vi "Main-loop.vi"() -> ()   [LabVIEW 2016]
uses:
  Sched_state.ctl
  Plant_info.ctl
  <vilib>/Platform/TimedLoop/XDataNode/timing_clust.ctl
  <vilib>/Platform/TimedLoop/XDataNode/nitl_modes.ctl
  <vilib>/Platform/TimedLoop/XDataNode/wakeup.ctl
  <vilib>/Platform/TimedLoop/XDataNode/XDataNode.xnode
  <vilib>/Platform/TimedLoop/XDataNode/XDNodeRunTimeDep.lvlib
panel:
  in  "Machine 1 IP Address":string="193.0.0.2"
  in  "Machine 2 IP address":string="193.0.0.4"
  in  "Plant 2 VI path":path=path "C:/ni-rt/startup/Plant2.vi"
  in  "Plant 1 VI path":path=path "C:/ni-rt/startup/Plant1.vi"
  out "error out":errorcluster
  out "loop time\n(only for diagnostics) - should be exactly 10, always":u32
  out "Plant 2 region":dbl(graph)
  out "Plant 1 region":dbl(graph)
  out "Plant 2":cluster{"Input":dbl, "Data":dbl, "Data":dbl}(graph)
  out "Plant 1":cluster{"Input":dbl, "Data":dbl, "Data":dbl}(graph)
  in  "error in (no error)":errorcluster
  in  "stop main":bool
  # "IMPORTANT! Deploy all files on the PXI machines in which the plants reside (Right-click on the target in the project > Deploy All) before starting this VI"
  # "Note that the \"VI paths\" for the plants refer to paths in the context of the respective PXI machines. not on this machine"
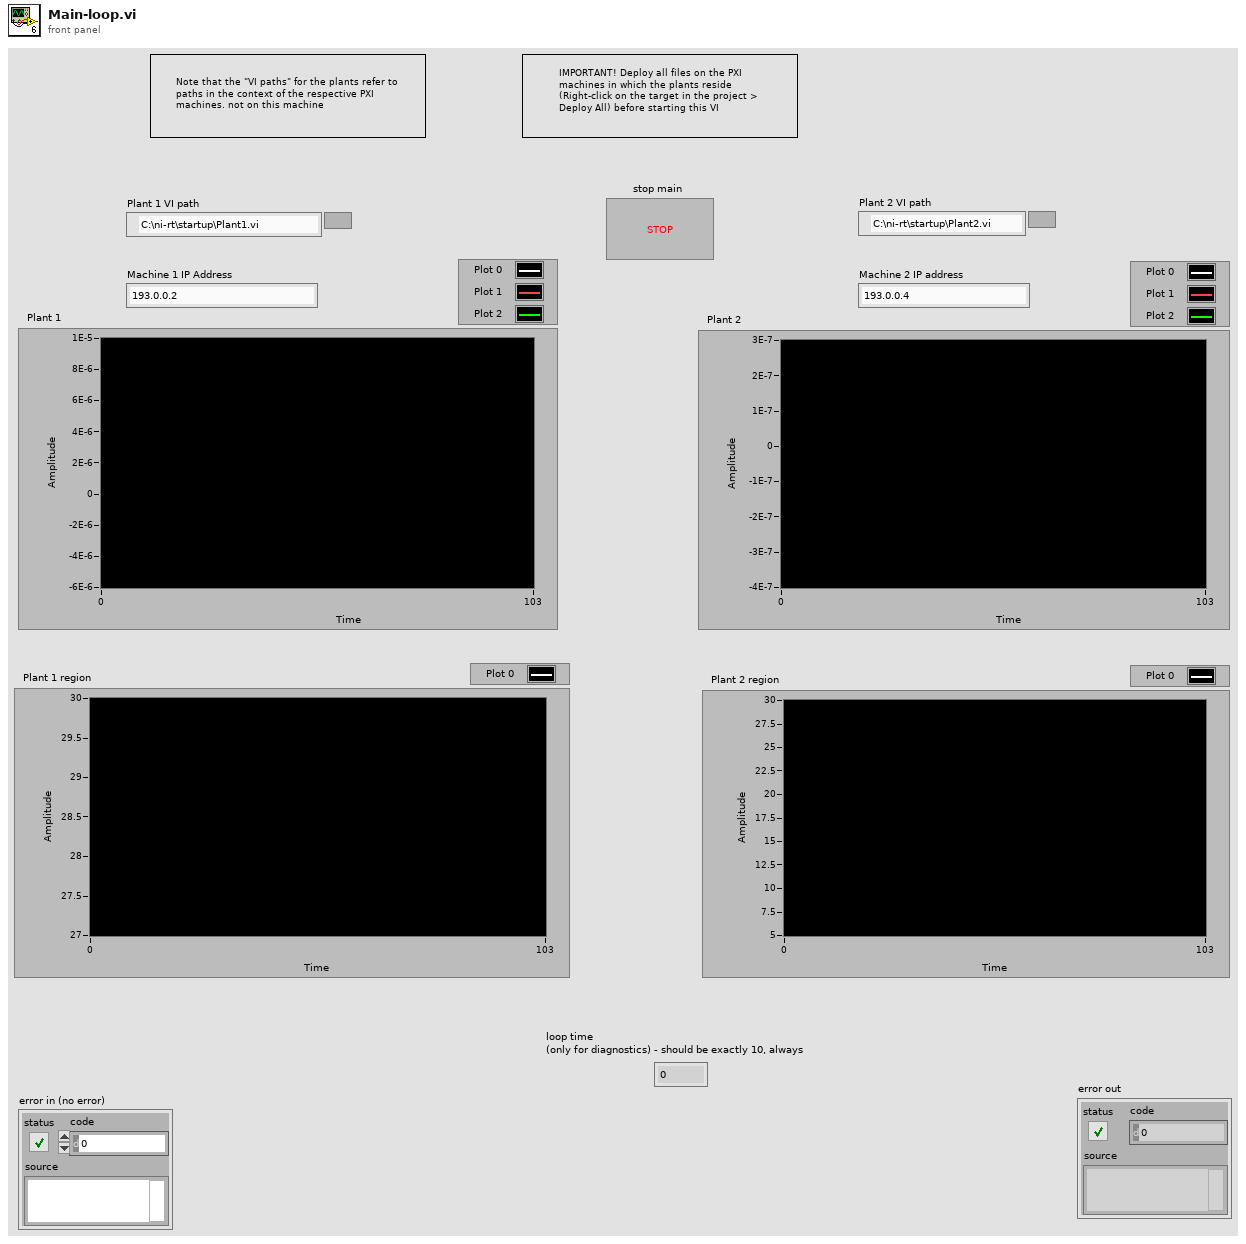
[diagram p1: front panel]
types:
  T1 = typedef "Sched_state.ctl" = cluster{"Plant 1":T2, "Plant 2":T2}
  T2 = typedef "Plant_info.ctl" = cluster{"Clk":dbl, "Region":dbl, "Input":dbl}
  T3 = typedef "Strategy_regional_cluster.ctl" = cluster{"Regional set array":T4[]}
  T4 = typedef "Strategy_regional_set.ctl" = cluster{"Lower lim":i32, "Upper lim":i32, "Equality req":i32, "First loop":i32, "Diff value":i32, "Trigg plant":i32}
  T5 = typedef "Plant-data.ctl" = cluster{"Plant X1 ":dbl[], "Plant X2":dbl[], "Plant K*x_hat":dbl[], "Region":i32[], "Trigger":i32[], "Early Trigg":i32[]}
  T6 = typedef "XDNodeRunTimeDep.lvlib/timing_clust.ctl" = cluster{"Expected End [f-1]":u64, "Actual End [f-1]":u64, "Finished Late? [f-1]":bool, "Expected End [i-1]":u64, "Actual End [i-1]":u64, "Finished Late? [i-1]":bool, "Expected Start [i]":u64, "Actual Start [i]":u64, "Expected Start [f]":u64, "Actual Start [f]":u64, "Source Name":string, "Structure Name":string, "Period":i64, "Deadline":i64, "Offset":i64, "Start":i64, "Priority":i32, "Timeout":i32, "Mode":T7, "Wakeup Reason":T8, "Error":errorcluster, "Source Type":string, "Secondary Source Type":string, "Global End Time":u64, "Global Start Time":u64, "Frame Duration":u64, "Iteration Duration":u64, "Assigned CPU":i32, "I/O Scan Engine Mode":u32}
  T7 = typedef "XDNodeRunTimeDep.lvlib/nitl_modes.ctl" = enum32{"No Change", "Process missed periods, maintain original phase", "Discard missed periods, maintain original phase", "Process missed periods, ignore original phase", "Discard missed periods, ignore original phase"}
  T8 = typedef "XDNodeRunTimeDep.lvlib/wakeup.ctl" = enum32{"Normal", "Aborted", "Asynchronous wakeup", "Timing source error", "Timed loop error", "Timeout"}
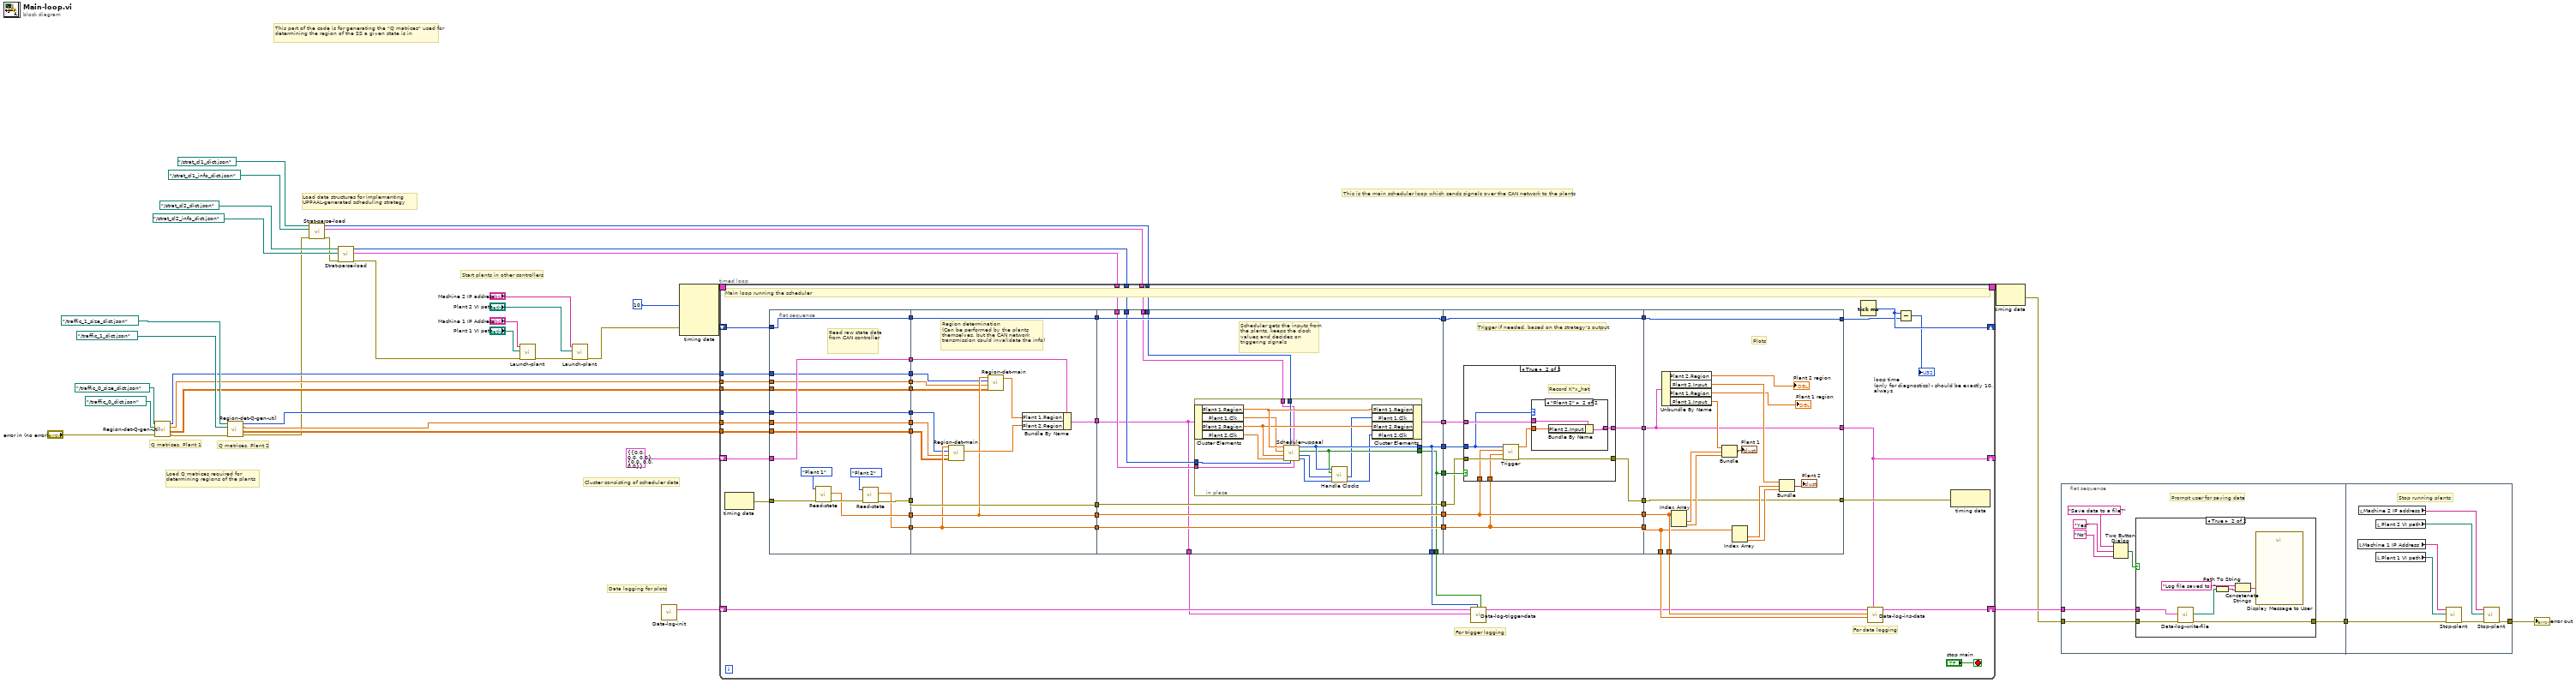
[diagram p0: block diagram]
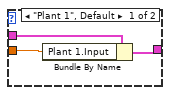
[diagram p4: hidden frame]
diagram:
  # "Load data structures for implementing UPPAAL-generated scheduling strategy"
  # "Load Q matrices required for determining regions of the plants"
  # "Data logging for plots"
  # "Q matrices, Plant 2"
  # "Q matrices, Plant 1"
  # "Cluster consisting of scheduler data"
  # "This part of the code is for generating the \"Q matrices\" used for determining the region of the SS a given state is in"
  # "Start plants in other controllers"
  # "This is the main scheduler loop which sends signals over the CAN network to the plants"
  n1 = call "Region-det-Q-gen-util.vi"("error in"="error in (no error)", "Actual Q matrix JSON - rel path"=path "../traffic_0_dict.json", "Q matrix info JSON - rel path"=path "../traffic_0_size_dict.json") -> ("error out"=w31:errorcluster, "Q Matrices"=w25:dbl[][][][], "Index array"=w26:dbl[], "Regions"=w27:i32[])  [unwired: 5 in]
  n2 = call "Region-det-Q-gen-util.vi"("error in"=w31, "Actual Q matrix JSON - rel path"=path "../traffic_1_dict.json", "Q matrix info JSON - rel path"=path "../traffic_1_size_dict.json") -> ("error out"=w15:errorcluster, "Q Matrices"=w28:dbl[][][][], "Index array"=w24:dbl[], "Regions"=w29:i32[])  [unwired: 5 in]
  n3 = call "Strat-parse-load.vi"("error in"=w15, "Info JSON - rel path"=path "../strat_cl1_info_dict.json", "Strategy JSON - rel path"=path "../strat_cl1_dict.json") -> ("error out"=w16:errorcluster, "Regional clusters"=w10:T3[], "Index array"=w11:i32[])  [unwired: 6 in]
  n4 = call "Strat-parse-load.vi"("error in"=w16, "Info JSON - rel path"=path "../strat_cl2_info_dict.json", "Strategy JSON - rel path"=path "../strat_cl2_dict.json") -> ("error out"=w7:errorcluster, "Regional clusters"=w13:T3[], "Index array"=w12:i32[])  [unwired: 6 in]
  n5 = call "Launch-plant.vi"("error in (no error)"=w7, "Plant VI path"="Plant 1 VI path", "Machine IP Address"="Machine 1 IP Address") -> ("error out"=w6:errorcluster)  [unwired: 7 in, 1 out]
  n6 = call "Launch-plant.vi"("error in (no error)"=w6, "Plant VI path"="Plant 2 VI path", "Machine IP Address"="Machine 2 IP address") -> ("error out"=w5:errorcluster)  [unwired: 7 in, 1 out]
  n7 = call "Data-log-init.vi"() -> ("Data cluster"=w23:cluster{"Plant 1":T5, "Plant 2":T5})  [unwired: 10 in, 1 out]
  n8 = node-c288(i64 10 ("Period"), w5) -> (w38:T6)  [unwired: 3 in]
  n9 = timed-loop {
    timing: w38 -> [_]
    timing-out: [_] -> w37
    shift-right: [w48] -> _
    shift-left: T1 {"Plant 1"={"Clk"=0.0, "Region"=0.0, "Input"=0.0}, "Plant 2"={"Clk"=0.0, "Region"=0.0, "Input"=0.0}} ("Scheduler State") -> [w90]
    tunnel: w29 -> [w72]
    tunnel: w24 -> [w69]
    tunnel: w28 -> [w67]
    tunnel: w27 -> [w65]
    tunnel: w26 -> [w64]
    tunnel: w25 -> [w61]
    shift-right: [w59] -> _
    shift-left: _ -> [w57]
    shift-right: [w51] -> w22
    shift-left: w23 -> [w43]
    tunnel: w13 -> [w47]
    tunnel: w12 -> [w46]
    tunnel: w11 -> [w45]
    tunnel: w10 -> [w44]
    stop <- "stop main" stop-if-true
    # "For trigger logging"
    # "For data logging"
    # "Main loop running the scheduler"
    n10 = node-c288() -> (w93:errorcluster)  [unwired: 1 in]
    n11 = flat-sequence {
      tunnel: w93 -> [w106]
      tunnel: w90 -> [w103]
      tunnel: [w103] -> w81
      tunnel: [w104] -> w77
      tunnel: [w102] -> w74
      tunnel: [w101] -> w73
      tunnel: w72 -> [w100]
      tunnel: [w100] -> w71
      tunnel: [w99] -> w70
      tunnel: w69 -> [w99]
      tunnel: [w98] -> w68
      tunnel: w67 -> [w98]
      tunnel: [w97] -> w66
      tunnel: w65 -> [w97]
      tunnel: w64 -> [w96]
      tunnel: [w96] -> w63
      tunnel: w61 -> [w95]
      tunnel: [w95] -> w62
      tunnel: w57 -> [w94]
      tunnel: [w94] -> w56
      tunnel: [w117] -> w87
      tunnel: [w116] -> w84
      tunnel: w81 -> [w122]
      tunnel: [w119] -> w80
      tunnel: [w118] -> w78
      tunnel: w77 -> [w118]
      tunnel: w74 -> [w117]
      tunnel: w73 -> [w116]
      tunnel: w71 -> [w115]
      tunnel: w70 -> [w114]
      tunnel: w68 -> [w113]
      tunnel: w66 -> [w112]
      tunnel: w63 -> [w110]
      tunnel: w62 -> [w111]
      tunnel: w56 -> [w109]
      tunnel: [w109] -> w55
      tunnel: [w124] -> w89
      tunnel: [w123] -> w88
      tunnel: w87 -> [w134]
      tunnel: [w134] -> w86
      tunnel: [w133] -> w85
      tunnel: w84 -> [w133]
      tunnel: [w132] -> w82
      tunnel: w80 -> [w125]
      tunnel: [w131] -> w79
      tunnel: w78 -> [w131]
      tunnel: w55 -> [w130]
      tunnel: [w130] -> w53
      tunnel: w47 -> [w129]
      tunnel: w46 -> [w128]
      tunnel: w45 -> [w127]
      tunnel: w44 -> [w126]
      tunnel: [w125] -> w41
      tunnel: [w124] -> w40
      tunnel: [w123] -> w39
      tunnel: [w154] -> w92
      tunnel: w89 -> [w150]
      tunnel: w88 -> [w155]
      tunnel: w86 -> [w152]
      tunnel: w85 -> [w151]
      tunnel: [w156] -> w83
      tunnel: w82 -> [w157]
      tunnel: w79 -> [w153]
      tunnel: [w151] -> w76
      tunnel: [w152] -> w75
      tunnel: [w149] -> w54
      tunnel: w53 -> [w149]
      tunnel: w92 -> [w178]
      tunnel: [w177] -> w48
      tunnel: w83 -> [w177]
      tunnel: w76 -> [w174]
      tunnel: w75 -> [w175]
      tunnel: [w178] -> w60
      tunnel: [w176] -> w58
      tunnel: w54 -> [w176]
      tunnel: [w175] -> w50
      tunnel: [w174] -> w49
      frame #0 {
        # "Read raw state data from CAN controller"
        n12 = call "Read-state.vi"("error in (no error)"=w106, "Plant"=enum16{"Plant 1", "Plant 2"}."Plant 1") -> ("error out"=w105:errorcluster, "state"=w102:dbl[])  [unwired: 8 in]
        n13 = call "Read-state.vi"("error in (no error)"=w105, "Plant"=enum16{"Plant 1", "Plant 2"}."Plant 2") -> ("error out"=w104:errorcluster, "state"=w101:dbl[])  [unwired: 8 in]
      }
      frame #1 {
        # "Region determination \n(Can be performed by the plants\nthemselves, but the CAN network \ntransmission could invalidate the info)"
        n14 = call "Region-det-main.vi"("Q Matrices"=w113, "Index Array"=w114, "Regions"=w115, "State"=w116) -> ("Region"=w120:dbl)  [unwired: 7 in]
        n15 = call "Region-det-main.vi"("Q Matrices"=w111, "Index Array"=w110, "Regions"=w112, "State"=w117) -> ("Region"=w121:dbl)  [unwired: 7 in]
        n16 = Bundle By Name(cluster=w122, "Plant 1.Region"=w121, "Plant 2.Region"=w120) -> (w119:T1)
      }
      frame #2 {
        # "Scheduler gets the inputs from the plants, keeps the clock values and decides on triggering signals"
        n17 = in-place {
          in-place-border: [w142] -> w124
          in-place-border: [w141] -> w123
          in-place-border: w129 -> [w146]
          in-place-border: w128 -> [w145]
          in-place-border: w127 -> [w144]
          in-place-border: w126 -> [w143]
          n18 = in-place-cluster #1(w125) -> ("Plant 1.Region"=w148:dbl, "Plant 1.Clk"=w135:dbl, "Plant 2.Region"=w147:dbl, "Plant 2.Clk"=w136:dbl)
          n19 = call "Scheduler-uppaal.vi"("Regional clusters, CL2"=w146, "Regional clusters, CL1"=w143, "Index array, CL2"=w145, "Index array, CL1"=w144, "Clock, plant 2"=w136, "Region, plant 2"=w147, "Clock, plant 1"=w135, "Region, plant 1"=w148) -> ("Clock 2"=w139:i32, "Clock 1"=w140:i32, "Trigger?"=w141:bool, "Plant to trigg"=w142:enum16{"Plant 1", "Plant 2"})
          n20 = call "Handle Clocks.vi"("CL2 Clock"=w139, "CL1 Clock"=w140, "Trigger?"=w141, "Plant to trigg"=w142) -> ("CL2 Clock"=w137:i32, "CL1 Clock"=w138:i32)  [unwired: 6 in]
          n21 = in-place-cluster #1("Plant 1.Region"=w148, "Plant 1.Clk"=w138, "Plant 2.Region"=w147, "Plant 2.Clk"=w137) -> (w132:T1)
        }
      }
      frame #3 {
        # "Trigger if needed, based on the strategy's output"
        n22 = case shown="True" w155 {
          tunnel: w157 -> [w159 w164]
          tunnel: [w159 w165] -> w156
          tunnel: w152 -> [_ w161]
          tunnel: w153 -> [w158 w167]
          tunnel: [w158 w166] -> w154
          tunnel: w150 -> [_ w163]
          tunnel: w151 -> [_ w160]
          frame False {
          }
          frame True {
            # "Record K*x_hat"
            n23 = call "Trigger.vi"("error in (no error)"=w167, "State, Plant 2"=w160, "State, Plant 1"=w161, "Plant to trigg"=w163) -> ("error out"=w166:errorcluster, "Kx"=w162:dbl)  [unwired: 6 in]
            n24 = case shown="\"Plant 2\"" w163 {
              tunnel: [w168 w173] -> w165
              tunnel: w164 -> [w170 w172]
              tunnel: w162 -> [w169 w171]
              frame "Plant 1", Default {
                n25 = Bundle By Name(cluster=w170, "Plant 1.Input"=w169) -> (w168:T1)
              }
              frame "Plant 2" {
                n26 = Bundle By Name(cluster=w172, "Plant 2.Input"=w171) -> (w173:T1)
              }
            }
          }
        }
      }
      frame #4 {
        # "Plots"
        n27 = Unbundle By Name(w177) -> ("Plant 2.Region"=→"Plant 2 region":dbl, "Plant 2.Input"=w184:dbl, "Plant 1.Region"=→"Plant 1 region":dbl, "Plant 1.Input"=w183:dbl)
        n28 = Index Array(array=w175) -> (element #1=w188:dbl, element #2=w187:dbl)  [unwired: 2 in]
        n29 = Bundle("Input"=w183, "Data"=w188, "Data"=w187) -> (→"Plant 1":cluster{"Input":dbl, "Data":dbl, "Data":dbl})  [unwired: 1 in]
        n30 = Index Array(array=w174) -> (element #1=w186:dbl, element #2=w185:dbl)  [unwired: 2 in]
        n31 = Bundle("Input"=w184, "Data"=w186, "Data"=w185) -> (→"Plant 2":cluster{"Input":dbl, "Data":dbl, "Data":dbl})  [unwired: 1 in]
      }
    }
    n32 = call "Data-log-trigger-data.vi"("Trigg?"=w39, "Plant to trigg"=w40, "Scheduler State"=w41, "Data cluster in"=w43) -> ("Data cluster out"=w42:cluster{"Plant 2":T5, "Plant 1":T5})  [unwired: 7 in]
    n33 = Tick Count (ms)() -> (millisecond timer value=w59:u32)
    n34 = call "Data-log-ins-data.vi"("Scheduler State"=w48, "Plant 2 State"=w49, "Plant 1 State"=w50, "Data cluster in"=w42) -> ("Data cluster out"=w51:cluster{"Plant 2":T5, "Plant 1":T5})  [unwired: 7 in]
    n35 = Subtract(x=w59, y=w58) -> (x-y=→"loop time\n(only for diagnostics) - should be exactly 10, always":u32)
    n36 = node-c288(w60) -> ()  [unwired: 1 out]
  }
  n37 = node-c288(w37) -> (w21:errorcluster)
  n38 = flat-sequence {
    tunnel: w22 -> [w200]
    tunnel: w21 -> [w199]
    tunnel: [w198] -> w2
    tunnel: w2 -> [w210]
    tunnel: [w209] -> w1
    frame #0 {
      # "Prompt user for saving data"
      n39 = Two Button Dialog(message="Save data to a file?", 1:"No" ("F button name (\"Cancel\")"), 2:"Yes" ("T button name (\"OK\")")) -> (T button?=w194:bool)
      n40 = case shown="True" w194 {
        tunnel: w200 -> [_ w207]
        tunnel: w199 -> [w201 w206]
        tunnel: [w201 w208] -> w198
        frame False {
        }
        frame True {
          n41 = call "Data-log-write-file.vi"("error in (no error)"=w206, "Data cluster in"=w207) -> ("error out"=w208:errorcluster, "new file path"=w205:path)  [unwired: 8 in]
          n42 = Path To String(path=w205) -> (string=w203:string)
          n43 = Concatenate Strings("Log file saved to: ", w203) -> (w202:string)
          n44 = call "Display Message to User"("Message"=w202) -> ()  [unwired: 9 in, 2 out]
        }
      }
    }
    frame #1 {
      # "Stop running plants"
      n45 = local read "Machine 1 IP Address"() -> (w213:string)
      n46 = local read "Machine 2 IP address"() -> (w215:string)
      n47 = local read "Plant 2 VI path"() -> (w214:path)
      n48 = local read "Plant 1 VI path"() -> (w212:path)
      n49 = call "Stop-plant.vi"("error in (no error)"=w210, "Plant VI path"=w212, "Machine IP Address"=w213) -> ("error out"=w211:errorcluster)  [unwired: 8 in]
      n50 = call "Stop-plant.vi"("error in (no error)"=w211, "Plant VI path"=w214, "Machine IP Address"=w215) -> ("error out"=w209:errorcluster)  [unwired: 8 in]
    }
  }
  "error out" <- w1
